vi "Write Command.vi"(4 "Instance":i32=1, 6 "Commands":T1=enum."Temp Feedback", 8 "error in (no error)":errorcluster, 10 "Set Value":string, 11 "Watlow F4T In":refnum<class "Watlow F4T.lvclass">) -> (0 "error out":errorcluster, 3 "Watlow F4T out":refnum<class "Watlow F4T.lvclass">)   [LabVIEW 2024, in "Watlow F4T.lvclass"]
uses:
  Watlow F4T.lvclass
  Private/Controls/Standard Bus Commands--Enum.ctl
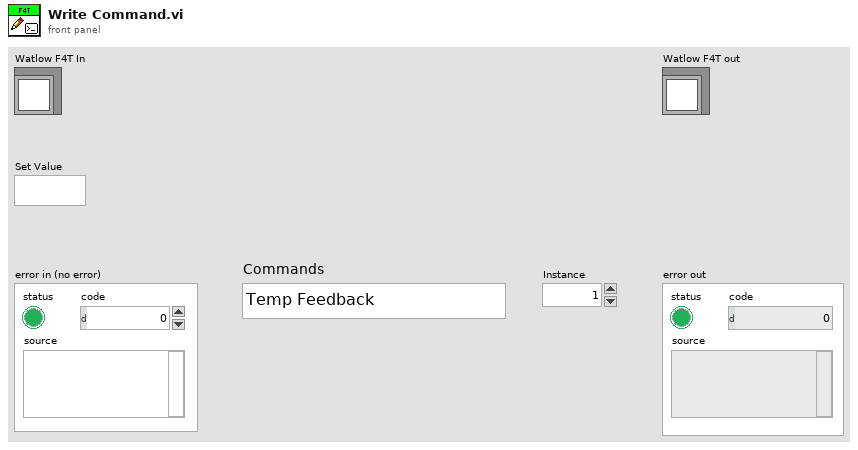
[diagram p1: front panel]
types:
  T1 = typedef "Watlow F4T.lvclass/Standard Bus Commands--Enum.ctl" = enum16{"Remote Setpoint", "Remote Mode", "Temp Feedback", "Target Setpoint", "Current Setpoint", "Setpoint Lower Limit", "Setpoint Upper Limit", "Ramp Rate Y", "Ramp Rate X", "Ramp Rate Action", "Temp Control State", "Temp Control Mode", "Power", "Heat Power", "Cool Power"}
  T2 = typedef "Watlow F4T.lvclass/Standard Bus Register LUT Data--Cluster.ctl" = cluster{"Parameter ID":i32, "Instance ID":i32}
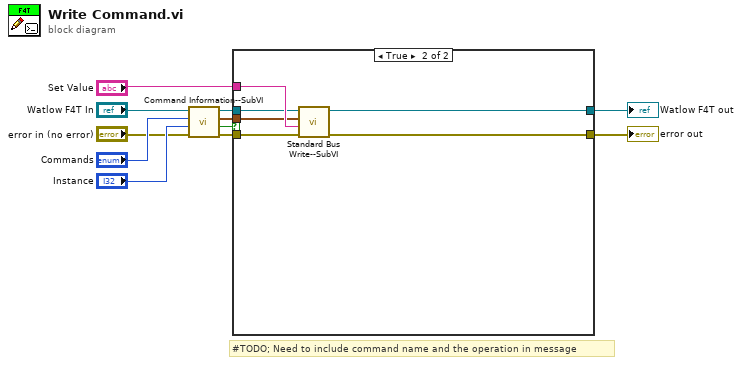
[diagram p0: block diagram]
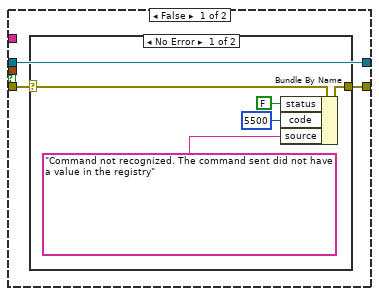
[diagram p2: hidden frame]
diagram:
  # "#TODO; Need to include command name and the operation in message"
  n1 = call "Command Information--SubVI.vi"("error in (no error)"="error in (no error)", "Instance"="Instance", "Commands"="Commands", "Watlow F4T In"="Watlow F4T In") -> ("error out"=w7:errorcluster, "Found?"=w3:bool, "Register"=w2:T2, "Watlow F4T Out"=w8:refnum<class "Watlow F4T.lvclass">)  [unwired: 4 in]
  n2 = case shown="True" w3 {
    tunnel: w7 -> [w14 w25]
    tunnel: w8 -> [w12 w22]
    tunnel: [w13 w26] -> w9
    tunnel: "Set Value" -> [_ w24]
    tunnel: w2 -> [_ w23]
    tunnel: [w12 w21] -> w1
    frame False {
      n3 = case shown="No Error" w14 {
        selector: w14 -> [w19 w20]
        tunnel: [w15 w20] -> w13
        frame No Error {
          n4 = Bundle By Name(cluster=w19, "status"=FALSE, "code"=5500, "source"="Command not recognized. The command sent did not have a value in the registry") -> (w15:errorcluster)
        }
        frame Error {
        }
      }
    }
    frame True {
      n5 = call "Standard Bus Write--SubVI.vi"("error in"=w25, "Set Value"=w24, "Register"=w23, "Watlow F4T in"=w22) -> ("error out"=w26:errorcluster, "Watlow F4T out"=w21:refnum<class "Watlow F4T.lvclass">)  [unwired: 6 in]
    }
  }
  "error out" <- w9
  "Watlow F4T out" <- w1
